vi "FindValidBuildSpecs.vi"(8 "error in (no error)":errorcluster, 9 "Target Name":string, 10 "ProjectItem Refnums":refnum<vi>[](array[refnum]), 11 "ExecuteMultipleBuildSpecs in":refnum<class "ExecuteMultipleBuildSpecs.lvclass">) -> (0 "error out":errorcluster, 1 "Specs":T1[](array[typedef]), 2 "dup ProjectItem Refnums":refnum<vi>[](array[refnum]), 3 "ExecuteMultipleBuildSpecs out":refnum<class "ExecuteMultipleBuildSpecs.lvclass">)   [LabVIEW 2014, in "ExecuteMultipleBuildSpecs.lvclass"]
uses:
  ExecuteMultipleBuildSpecs.lvclass
  SpecInformation.ctl
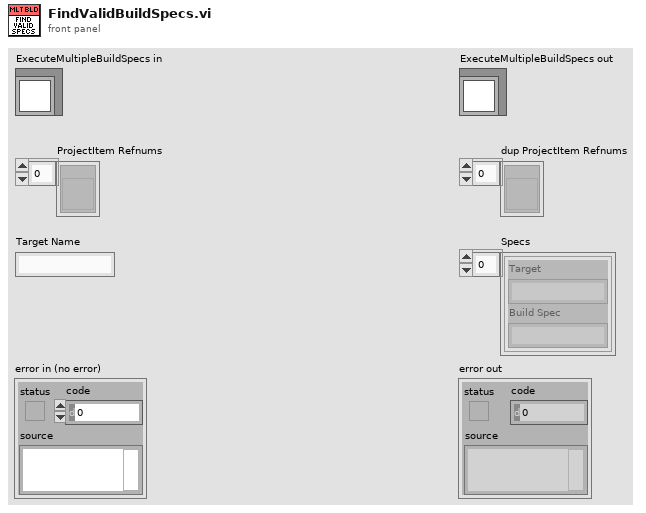
[diagram p1: front panel]
types:
  T1 = typedef "ExecuteMultipleBuildSpecs.lvclass/SpecInformation.ctl" = cluster{"Target":string, "Build Spec":string}
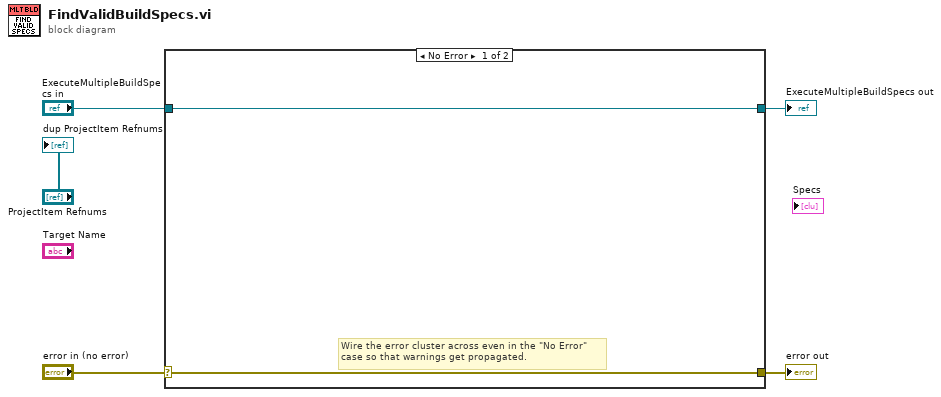
[diagram p0: block diagram]
diagram:
  n1 = case shown="No Error" "error in (no error)" {
    selector: "error in (no error)" -> [w6 w9]
    tunnel: [w6 w9] -> w4
    tunnel: [w7 w8] -> w2
    tunnel: "ExecuteMultipleBuildSpecs in" -> [w7 w8]
    frame No Error {
      # "Wire the error cluster across even in the \"No Error\"\ncase so that warnings get propagated."
    }
    frame Error {
    }
  }
  "error out" <- w4
  "ExecuteMultipleBuildSpecs out" <- w2
  "dup ProjectItem Refnums" <- "ProjectItem Refnums"
